vi "PH_Img_BaseClass.set Notifier.vi"(0 "i ref in":refnum<vi>, 5 "error in":errorcluster) -> (14 "i ref out":refnum<vi>, 19 "error out":errorcluster)   [LabVIEW 2014, in "PH_Img_BaseClass.lvlib"]
uses:
  PH_Img_BaseClass.lvlib
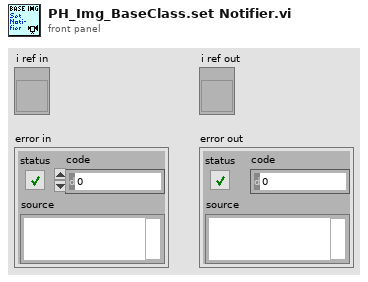
[diagram p1: front panel]
types:
  T1 = typedef "PH_Img_BaseClass.lvlib/PH_Img_BaseClass.i attribute.ctl" = cluster{"GUI Refs":T2, "Timeout Image [ms]":i32, "Default Periodic Period [ms]":i32, "Camera":cluster{"Instancename":string, "Notifier":refnum<notifier>}, "Palette":T3, "Cam Settings":cluster{"Cam ID":string, "Gain":dbl, "Brightness":dbl, "Shutter":dbl, "Cam Info Failure":bool, "Mode":i32}}
  T2 = typedef "PH_Img_BaseClass.lvlib/PH_Img_BaseClass.GUI Refs.ctl" = cluster{"Timeout":refnum<vi>, "Image":refnum<vi>, "Palette":refnum<vi>, "Timeout Set":refnum<vi>}
  T3 = typedef "PH_Img_BaseClass.lvlib/PH_Img_BaseClass.Palette.ctl" = i32
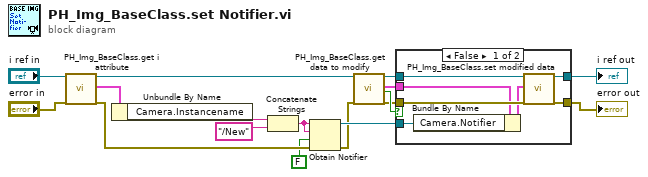
[diagram p0: block diagram]
diagram:
  n1 = call "PH_Img_BaseClass.get i attribute.vi"("i ref in"="i ref in", "error in (no error)"="error in") -> ("i ref out"=w13:refnum<vi>, "i attribute"=w16:T1, "error out"=w15:errorcluster)  [unwired: 15 in]
  n2 = Unbundle By Name(w16) -> ("Camera.Instancename"=w17:string)
  n3 = Concatenate Strings(w17, "/New" ("name")) -> (w3:string)
  n4 = Obtain Notifier(name (unnamed)=w3, notification data type=w3, create if not found? (T)=FALSE ("return existing (F)"), error in (no error)=w15) -> (notifier out=w11:refnum<notifier>, error out=w8:errorcluster)  [unwired: 1 out]
  n5 = call "PH_Img_BaseClass.get data to modify.vi"("i ref in"=w13, "error in (no error)"=w8) -> ("i ref out"=w4:refnum<vi>, "i attribute"=w10:T1, "timed out"=w12:bool, "error out"=w7:errorcluster)  [unwired: 14 in]
  n6 = case shown="False" w12 {
    tunnel: w4 -> [w24 w26]
    tunnel: [w23 w26] -> w6
    tunnel: w7 -> [w22 w25]
    tunnel: [w21 w25] -> w9
    tunnel: w10 -> [w20 _]
    tunnel: w11 -> [w18 _]
    frame False {
      n7 = Bundle By Name(cluster=w20, "Camera.Notifier"=w18) -> (w19:T1)
      n8 = call "PH_Img_BaseClass.set modified data.vi"("i ref in"=w24, "i attribute"=w19, "error in (no error)"=w22) -> ("i ref out"=w23:refnum<vi>, "error out"=w21:errorcluster)  [unwired: 15 in]
    }
    frame True {
    }
  }
  "error out" <- w9
  "i ref out" <- w6
